vi "ADO Connection Check Table Exist.vi"(8 "error in (no error)":errorcluster caption="错误输入（无错误）", 9 "table name":string, 11 "Database Connection 输入":refnum<class "Database Connection.lvclass"> caption="DNL_LabVIEW Object in") -> (0 "error out":errorcluster caption="错误输出", 1 "Exists?":bool, 3 "Database Connection 输出":refnum<class "Database Connection.lvclass"> caption="DNL_LabVIEW Object out")   [LabVIEW 2011, in "Database Connection.lvclass"]
uses:
  Database Connection.lvclass
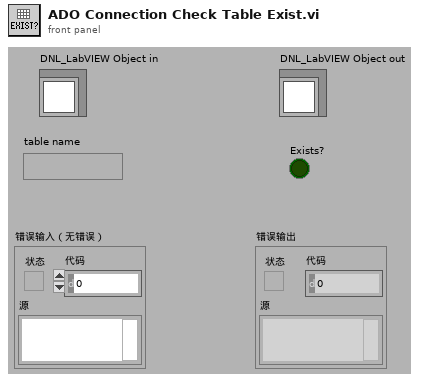
[diagram p1: front panel]
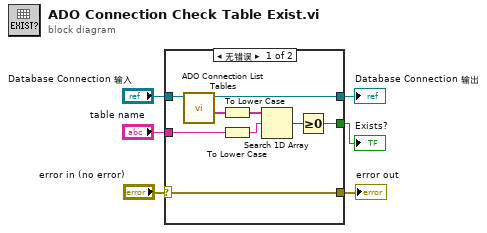
[diagram p0: block diagram]
diagram:
  n1 = case shown="无错误" "error in (no error)" {
    selector: "error in (no error)" -> [w15 w17]
    tunnel: [w15 w17] -> w5
    tunnel: [w13 w16] -> w3
    tunnel: "Database Connection 输入" -> [w14 w16]
    tunnel: "table name" -> [w8 _]
    tunnel: [w7 _] -> w1
    frame No Error {
      n2 = call "ADO Connection List Tables.vi"("Database Connection 输入"=w14) -> ("Tables"=w9:string[], "Database Connection 输出"=w13:refnum<class "Database Connection.lvclass">)  [unwired: 8 in, 1 out]
      n3 = To Lower Case(string=w9) -> (all lower case string=w11:string[])
      n4 = To Lower Case(string=w8) -> (all lower case string=w12:string)
      n5 = Search 1D Array(1D array=w11, element=w12) -> (index of element=w10:i32)  [unwired: 1 in]
      n6 = Greater Or Equal To 0?(x=w10) -> (x >= 0?=w7:bool)
    }
    frame Error {
    }
  }
  "error out" <- w5
  "Database Connection 输出" <- w3
  "Exists?" <- w1
